vi "GetCRefVariantInfo.vi"(2 "variant":variant) -> (16 "CRef Type":T1)   [LabVIEW 2012, in "CRef.lvlib"]
uses:
  Core/Master Types.ctl
  CRef.lvlib
  <vilib>/Utility/VariantDataType/VariantType.lvlib
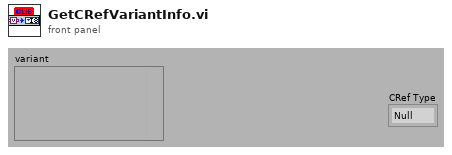
[diagram p1: front panel]
types:
  T1 = typedef "CRef.lvlib/Master Types.ctl" = enum8{"Null", "Boolean", "U8", "I8", "U16", "I16", "U32", "I32", "U64", "I64", "Single", "Double", "Extended", "CSG", "CDB", "CXT", "Boolean(Def)", "U8(Def)", "I8(Def)", "U16(Def)", "I16(Def)", "U32(Def)", "I32(Def)", "Reserved Def", "Reserved Def1", "Single(Def)", "Double(Def)", "Reserved Def2", "Reserved Def3", "Reserved Def4", "Reserved Def5", "Unsigned(Def)", "Signed(Def)", "Real(Def)", "Reserved Def6", "Numeric(Def)", "String"}
  T2 = typedef "VariantType.lvlib/Type.ctl" = enum8{"Invalid Type", "Void", "I8", "I16", "I32", "I64", "U8", "U16", "U32", "U64", "Single Float", "Double Float", "Extended Float", "Single Complex", "Double Complex", "Extended Complex", "Enum U8", "Enum U16", "Enum U32", "Enum U64", "Single Float With Unit", "Double Float With Unit", "Extended Float With Unit", "Single Complex with Unit", "Double Complex with Unit", "Extended Complex with Unit", "Boolean", "String", "Path", "Picture", "Tag", "Array", "Cluster", "Variant", "LV Variant", "Waveform", "Timestamp", "Digital Waveform", "Digital Data", "ExpressData", "Refnum", "External Data", "VI", "Poly VI", "LabVIEW Class Instance", "Fixed Point"}
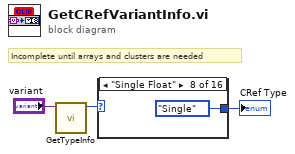
[diagram p0: block diagram]
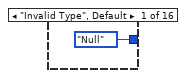
[diagram p2: hidden frame]
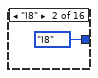
[diagram p3: hidden frame]
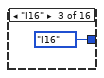
[diagram p4: hidden frame]
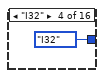
[diagram p5: hidden frame]
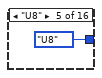
[diagram p6: hidden frame]
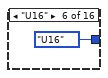
[diagram p7: hidden frame]
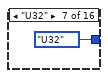
[diagram p8: hidden frame]
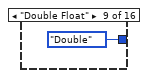
[diagram p9: hidden frame]
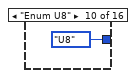
[diagram p10: hidden frame]
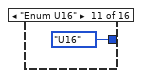
[diagram p11: hidden frame]
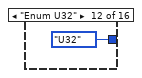
[diagram p12: hidden frame]
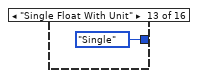
[diagram p13: hidden frame]
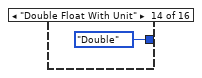
[diagram p14: hidden frame]
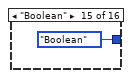
[diagram p15: hidden frame]
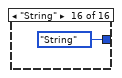
[diagram p16: hidden frame]
diagram:
  # "Incomplete until arrays and clusters are needed"
  n1 = call <vilib>:"GetTypeInfo.vi"("Variant"="variant") -> ("Type Enum"=w2:T2)  [unwired: 6 in, 4 out]
  n2 = case shown="\"Single Float\"" w2 {
    tunnel: [Master_Types."Null" ("CRef Type") Master_Types."I8" ("CRef Type") Master_Types."I16" ("CRef Type") Master_Types."I32" ("CRef Type") Master_Types."U8" ("CRef Type") Master_Types."U16" ("CRef Type") Master_Types."U32" ("CRef Type") Master_Types."Single" ("CRef Type") Master_Types."Double" ("CRef Type") Master_Types."U8" ("CRef Type") Master_Types."U16" ("CRef Type") Master_Types."U32" ("CRef Type") Master_Types."Single" ("CRef Type") Master_Types."Double" ("CRef Type") Master_Types."Boolean" ("CRef Type") Master_Types."String" ("CRef Type")] -> w1
    frame "Invalid Type", Default {
    }
    frame "I8" {
    }
    frame "I16" {
    }
    frame "I32" {
    }
    frame "U8" {
    }
    frame "U16" {
    }
    frame "U32" {
    }
    frame "Single Float" {
    }
    frame "Double Float" {
    }
    frame "Enum U8" {
    }
    frame "Enum U16" {
    }
    frame "Enum U32" {
    }
    frame "Single Float With Unit" {
    }
    frame "Double Float With Unit" {
    }
    frame "Boolean" {
    }
    frame "String" {
    }
  }
  "CRef Type" <- w1
